vi "USRP_v2.vi"() -> ()   [LabVIEW 2018]
uses:
  <instrlib>/niUSRP/niUSRP Timestamp.ctl
  <vilib>/addons/Modulation/niDMT.lvlib
  <vilib>/addons/Modulation/Digital/General/MT Apply Matched Filter (Generic).vi
  <instrlib>/niUSRP/niUSRP Write Tx Data (CDB Cluster).vi
  <instrlib>/niUSRP/niUSRP Fetch Rx Data (CDB Cluster).vi
  <instrlib>/niUSRP/niUSRP Configure Time Start Trigger.vi
panel:
  out "Y 3":cdb[](array[numeric])
  out "Y 2":cdb[](array[numeric])
  out "error out 3":errorcluster
  out "dec":i8[](array[numeric])
  out "IQ Constellation 2":T1(graph) caption="IQ Constellation"
  out "IQ Constellation":T1(graph)
  out "Y":cdb[](array[numeric])
  out "size(s)":i32
  out "Waveform Graph 2":dbl[](graph)
  out "error out 2":errorcluster
  in  "Enabled Channel 2":string(combo)="0"
  out "Coerced Gain 2":dbl format="%#_6f"
  in  "Active Antenna 2":string="TX1"
  in  "Stop 2":bool
  in  "Timeout 2":dbl=10.0
  out "Coerced Carrier Frequency 2":dbl=100000.0 format="%#_6p"
  out "Coerced IQ Rate 2":dbl=100000.0 format="%#_6p"
  in  "Gain 2":dbl format="%#_6f"
  in  "Carrier Frequency 2":dbl=2000000000.0 format="%#_6p"
  in  "IQ Rate 2":dbl=1000000.0 format="%#_6p"
  out "error out":errorcluster
  in  "Enabled Channel":string="0"
  in  "Number of Samples":i64=16384
  in  "Timeout":dbl=10.0
  out "Actual Rx Timestamp":T2
  in  "Time to Receive First Sample":T2={"whole seconds"=2, "fractional seconds"=0.0}
  in  "Active Antenna":string="RX1"
  out "Coerced Gain":dbl format="%#_6f"
  out "Coerced Carrier Frequency":dbl=100000.0 format="%#_6p"
  out "Coerced IQ Rate":dbl=100000.0 format="%#_6p"
  in  "Gain":dbl=1.0 format="%#_6f"
  in  "Carrier Frequency":dbl=2000000000.0 format="%#_6p"
  in  "IQ Rate":dbl=1000000.0 format="%#_6p"
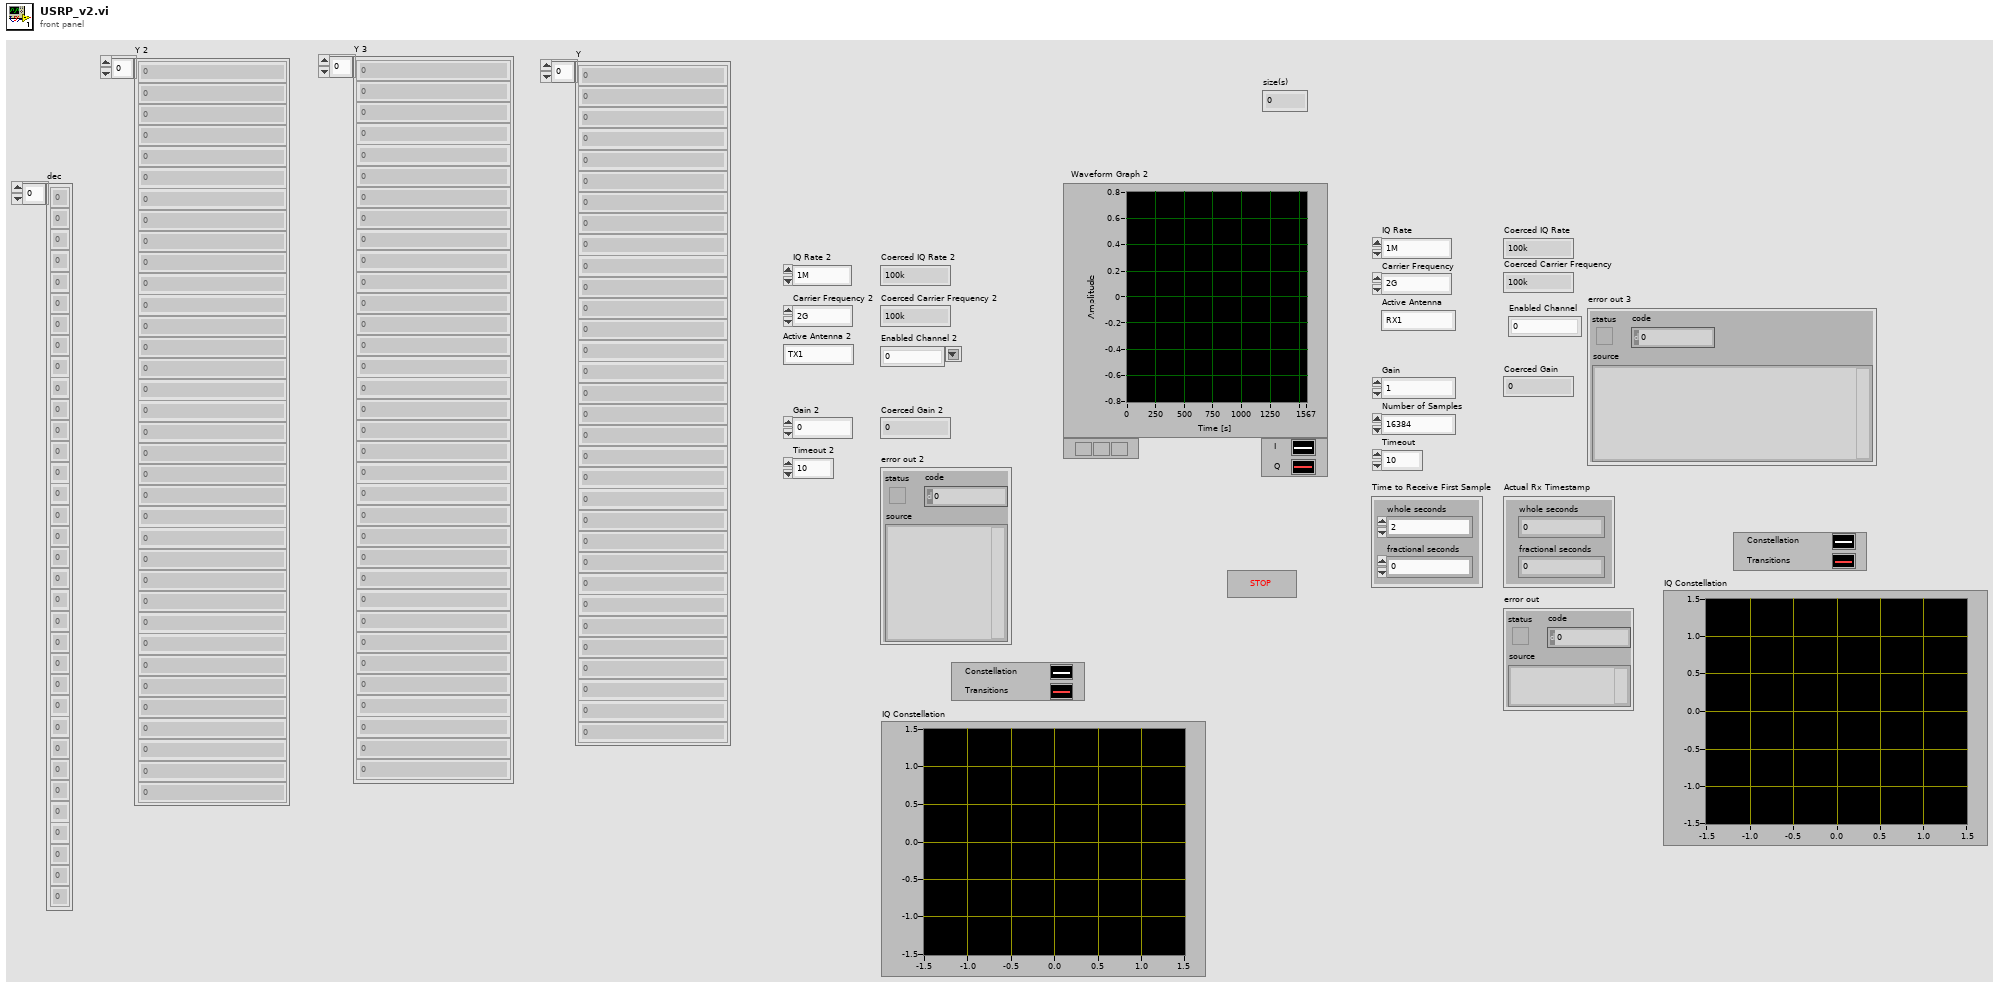
[diagram p1: front panel]
types:
  T1 = cluster{"Decimated Array":dbl[], "Decimated Array":dbl[]}[]
  T2 = typedef "niUSRP Timestamp.ctl" = cluster{"whole seconds":u64, "fractional seconds":dbl}
  T3 = enum16{"none", "Raised Cosine", "Root Raised Cos", "Gaussian"}
  T4 = typedef "niAMT.lvlib/Complex Data Waveform.ctl" = cluster{"t0":dbl, "dt":dbl, "Y":cdb[]}
  T5 = cluster{"constellation":dbl[], "oversampled data":dbl[]}[]
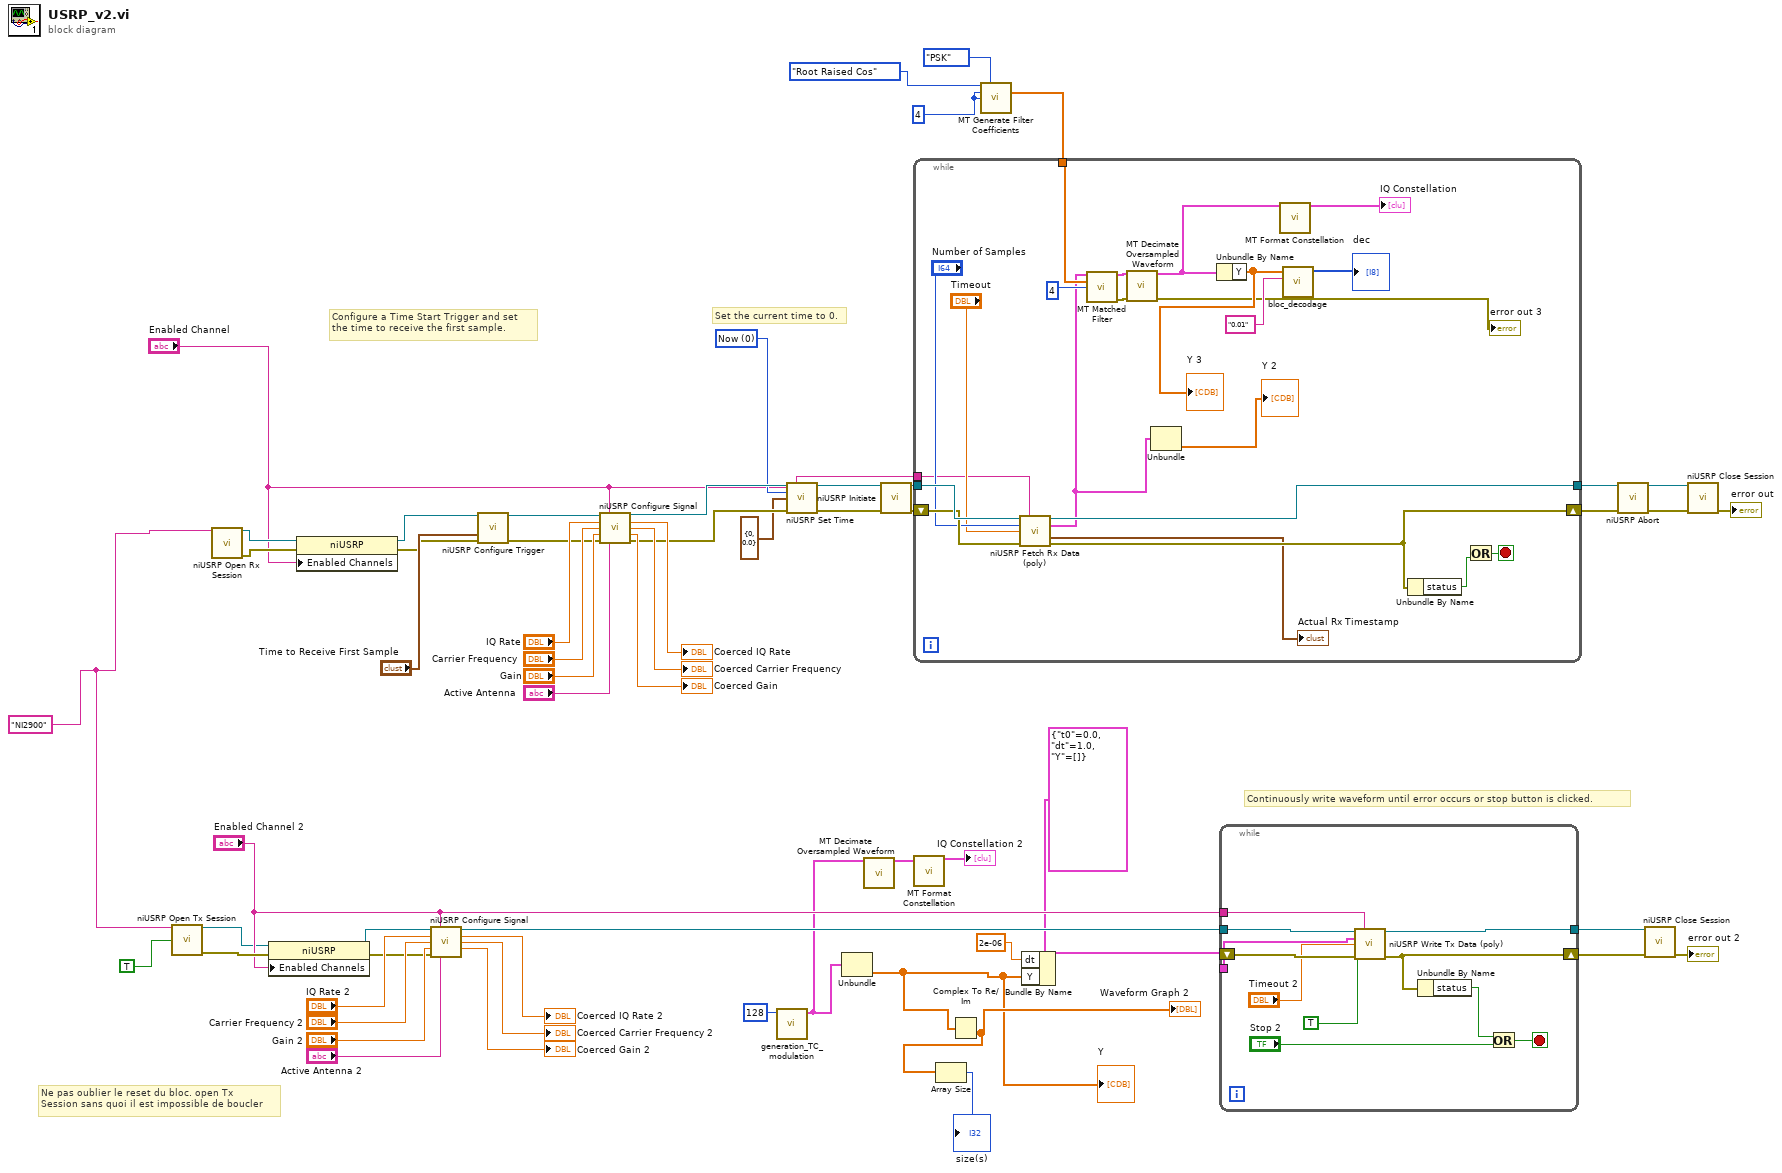
[diagram p0: block diagram]
diagram:
  w9 = 4 ("pulse shaping samples per symbol (16)")
  w19 = 0 items=["Now", "Next Timebase Edge"] ("when")
  w40 = "NI2900"
  # "Configure a Time Start Trigger and set \nthe time to receive the first sample."
  # "Set the current time to 0."
  # "Ne pas oublier le reset du bloc. open Tx \nSession sans quoi il est impossible de boucler"
  # "Continuously write waveform until error occurs or stop button is clicked."
  n1 = call <instrlib>:"niUSRP Open Tx Session.vi"("device names"=w40, "reset"=TRUE) -> ("session handle out"=w42:refnum<k15>, "error out"=w50:errorcluster)  [unwired: 12 in]
  n2 = call <instrlib>:"niUSRP Open Rx Session.vi"("device names"=w40) -> ("session handle out"=w17:refnum<k15>, "error out"=w15:errorcluster)  [unwired: 13 in]
  n3 = property class="niUSRP"(reference=w42, error in=w50, "Enabled Channels"="Enabled Channel 2") -> (reference out=w49:refnum<k15>, error out=w48:errorcluster)
  n4 = property class="niUSRP"(reference=w17, error in=w15, "Enabled Channels"="Enabled Channel") -> (reference out=w16:refnum<k15>, error out=w14:errorcluster)
  n5 = call <instrlib>:"niUSRP Configure Signal.vi"("session handle"=w49, "channel list"="Enabled Channel 2", "IQ rate"="IQ Rate 2", "carrier frequency"="Carrier Frequency 2", "gain"="Gain 2", "error in (no error)"=w48, "active antenna"="Active Antenna 2") -> ("session handle out"=w57:refnum<k15>, "coerced IQ rate"=→"Coerced IQ Rate 2":dbl, "coerced carrier frequency"=→"Coerced Carrier Frequency 2":dbl, "coerced gain"=→"Coerced Gain 2":dbl)  [unwired: 4 in, 1 out]
  n6 = call-poly <instrlib>:"niUSRP Configure Trigger.vi"("session handle"=w16, "start trigger time"="Time to Receive First Sample", "error in (no error)"=w14) -> ("session handle out"=w24:refnum<k15>, "error out"=w23:errorcluster)  [unwired: 11 in]
  n7 = call <instrlib>:"niUSRP Configure Signal.vi"("session handle"=w24, "channel list"="Enabled Channel", "IQ rate"="IQ Rate", "carrier frequency"="Carrier Frequency", "gain"="Gain", "error in (no error)"=w23, "active antenna"="Active Antenna") -> ("session handle out"=w26:refnum<k15>, "coerced IQ rate"=→"Coerced IQ Rate":dbl, "coerced carrier frequency"=→"Coerced Carrier Frequency":dbl, "coerced gain"=→"Coerced Gain":dbl, "error out"=w25:errorcluster)  [unwired: 4 in]
  n8 = call "generation_TC_modulation.vi"("Numeric"=128) -> ("output complex waveform"=w5:T4)  [unwired: 8 in, 2 out]
  n9 = call <instrlib>:"niUSRP Set Time.vi"("session handle"=w26, "channel list"="Enabled Channel", "apply timestamp"=w19, "timestamp"=T2 {"whole seconds"=0, "fractional seconds"=0.0} ("Time Now"), "error in (no error)"=w25) -> ("session handle out"=w21:refnum<k15>, "error out"=w20:errorcluster)  [unwired: 9 in]
  n10 = Unbundle(w5) -> ("Y"=w1:cdb[])  [unwired: 2 out]
  "Y" <- w1
  n11 = call <vilib>:"MT Decimate Oversampled Waveform.vi"("input complex waveform"=w5) -> ("output complex waveform"=w6:T4)  [unwired: 13 in, 1 out]
  n12 = call <instrlib>:"niUSRP Initiate.vi"("session handle"=w21, "error in (no error)"=w20) -> ("session handle out"=w39:refnum<k15>, "error out"=w38:errorcluster)  [unwired: 12 in]
  n13 = call <vilib>:"MT Format Constellation.vi"("waveform"=w6) -> ("constellation graph"=→"IQ Constellation 2":T5)  [unwired: 13 in, 1 out]
  n14 = Complex To Re/Im(x + iy=w1) -> (y=w41:dbl[])  [unwired: 1 out]
  "Waveform Graph 2" <- w41
  n15 = Array Size(array=w41) -> (size(s)=→"size(s)":i32)
  n16 = call <vilib>:"MT Generate Filter Coefficients.vi"("pulse shaping filter (none)"=T3."Root Raised Cos", "modulation type"=enum16{"FSK", "PSK", "QAM", "MSK", "PAM", "ASK"}."PSK", "pulse shaping samples per symbol (16)"=w9, "matched samples per symbol (16)"=w9) -> ("matched filter coefficients"=w8:dbl[])  [unwired: 9 in, 2 out]
  n17 = while {
    tunnel: w39 -> [w83]
    tunnel: [w79] -> w37
    shift-right: [w78] -> w36
    shift-left: w38 -> [w82]
    tunnel: "Enabled Channel" -> [w73]
    tunnel: w8 -> [w69]
    stop <- w77 stop-if-true
    n18 = call-poly <instrlib>:"niUSRP Fetch Rx Data (poly).vi"("session handle"=w83, "channel list"=w73, "number of samples"="Number of Samples", "timeout"="Timeout", "error in (no error)"=w82) -> ("session handle out"=w79:refnum<k15>, "data"=w62:cluster{"t0":dbl, "dt":dbl, "Y":cdb[]}, "timestamp"=→"Actual Rx Timestamp":T2, "error out"=w78:errorcluster)  [unwired: 7 in]
    n19 = call-poly <vilib>:"MT Matched Filter.vi"("input complex waveform"=w62, "matched filter coefficients"=w69, "samples per symbol (16)"=4) -> ("output complex waveform"=w71:T4, "error out"=w64:errorcluster)  [unwired: 11 in]
    n20 = call <vilib>:"MT Decimate Oversampled Waveform.vi"("input complex waveform"=w71, "error in (no error)"=w64) -> ("output complex waveform"=w66:T4, "error out"=→"error out 3":errorcluster)  [unwired: 12 in]
    n21 = Unbundle(w62) -> ("Y"=→"Y 2":cdb[])  [unwired: 2 out]
    n22 = Unbundle By Name(w66) -> ("Y"=w65:cdb[])
    "Y 3" <- w65
    n23 = call <vilib>:"MT Format Constellation.vi"("waveform"=w66) -> ("constellation graph"=→"IQ Constellation":T5)  [unwired: 13 in, 1 out]
    n24 = call "bloc_decodage.vi"("sigma2"="0.01", "Array"=w65) -> ("output bit stream"=→"dec":i8[])  [unwired: 7 in, 2 out]
    n25 = Unbundle By Name(w78) -> ("status"=w74:bool)
    n26 = Or(y=w74) -> (x=w75:bool, x .or. y?=w77:bool)
  }
  n27 = Bundle By Name(cluster=cluster{"t0":dbl, "dt":dbl, "Y":cdb[]} {"t0"=0.0, "dt"=1.0, "Y"=[]} ("data"), "dt"=2e-06, "Y"=w1) -> (w2:cluster{"t0":dbl, "dt":dbl, "Y":cdb[]})
  n28 = while {
    tunnel: w57 -> [w93]
    tunnel: [w90] -> w56
    shift-right: [w89] -> w55
    shift-left: _ -> [w92]
    tunnel: "Enabled Channel 2" -> [w86]
    tunnel: w2 -> [w84]
    stop <- w94 stop-if-true
    n29 = call-poly <instrlib>:"niUSRP Write Tx Data (poly).vi"("session handle"=w93, "channel list"=w86, "data"=w84, "timeout"="Timeout 2", "end of data?"=TRUE, "error in (no error)"=w92) -> ("session handle out"=w90:refnum<k15>, "error out"=w89:errorcluster)  [unwired: 8 in]
    n30 = Unbundle By Name(w89) -> ("status"=w88:bool)
    n31 = Or(x=w88, y="Stop 2") -> (x .or. y?=w94:bool)
  }
  n32 = call <instrlib>:"niUSRP Abort.vi"("session handle"=w37, "error in (no error)"=w36) -> ("session handle out"=w34:refnum<k15>, "error out"=w35:errorcluster)  [unwired: 12 in]
  n33 = call <instrlib>:"niUSRP Close Session.vi"("session handle"=w56, "error in (no error)"=w55) -> ("error out"=→"error out 2":errorcluster)  [unwired: 13 in]
  n34 = call <instrlib>:"niUSRP Close Session.vi"("session handle"=w34, "error in (no error)"=w35) -> ("error out"=→"error out":errorcluster)  [unwired: 13 in]
